vi "OAT LP Kaiser Window Design.vi"(8 "A stop [dB]":dbl=72.0 format="%.2f", 9 "stopband":dbl=0.25 format="%.2f", 10 "passband":dbl=0.05 format="%.2f", 11 "fs":dbl=1.0 format="%.2f") -> (0 "error":i32, 2 "taps":i32, 3 "filter coefficients":dbl[](array[numeric]) format="%.2f")   [LabVIEW 2017, in "SoundVib_Resampling.lvlib"]
uses:
  <vilib>/addons/Sound and Vibration/Order Analysis/Resample Order Tracking/SoundVib_Resampling.lvlib
  <vilib>/Analysis/4window.llb/windowTd.ctl
  <vilib>/Analysis/NI_AALBase.lvlib
  <vilib>/Analysis/NI_AALPro.lvlib
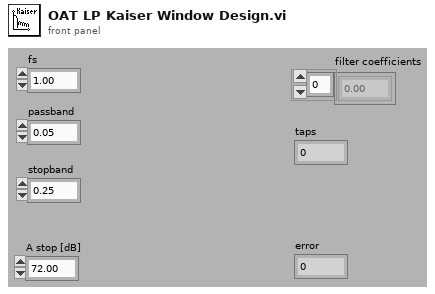
[diagram p1: front panel]
types:
  T1 = typedef "NI_AALPro.lvlib/windowTd.ctl" = u32
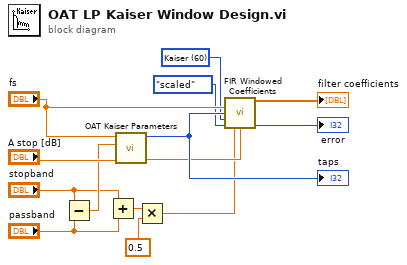
[diagram p0: block diagram]
diagram:
  w6 = T1 60 items=["Rectangle"=0, "Hanning"=1, "Hamming"=2, "Blackman-Harris"=3, "Exact Blackman"=4, "Blackman"=5, "Flat Top"=6, "4 Term B-Harris "=7, "7 Term B-Harris"=8, "Low Sidelobe"=9, "Blackman Nuttall"=11, "Triangle"=30, "Bartlett-Hanning"=31, "Bohman"=32, "Parzen"=33, "Welch"=34, "Kaiser"=60, "Dolph-Chebyshev"=61, "Gaussian"=62] ("window")
  n1 = Subtract(x="stopband", y="passband") -> (x-y=w13:dbl)
  n2 = Add(x="stopband", y="passband") -> (x+y=w9:dbl)
  n3 = call <vilib>:"OAT Kaiser Parameters.vi"("A stop [dB]"="A stop [dB]", "delta f"=w13, "fs"="fs") -> ("beta"=w4:dbl, "taps"=w7:i32)  [unwired: 7 in]
  "taps" <- w7
  n4 = Multiply(x=w9, y=0.5) -> (x*y=w3:dbl)
  n5 = call <vilib>:"FIR Windowed Coefficients.vi"("window parameter"=w4, "sampling freq: fs"="fs", "taps"=w7, "window"=w6, "option"=enum32{"not scaled", "scaled"}."scaled", "low cutoff freq: fl"=w3) -> ("FIR Windowed Coefficients"=→"filter coefficients":dbl[], "error"=→"error":i32)  [unwired: 8 in]
